vi "ERR Error Dialog.vi"(0 "Error Item":string, 9 "Description":string, 11 "Error In (no error)":errorcluster) -> ()   [LabVIEW 2011]
doc: "This is a 3-button dialog for the use of error handling such that a choice can be made by the user to either Recover from an error, pass the error through, or stop LabVIEW.\n\nThis vi was created by David Gianetto, contact me with any problems, questions, etc."
panel:
  out "Description Display":string
  in  "OK":bool
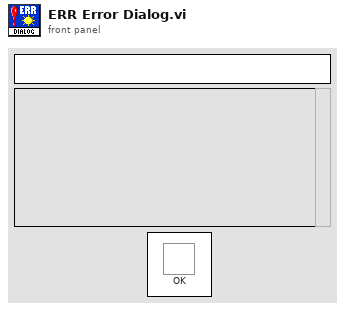
[diagram p1: front panel]
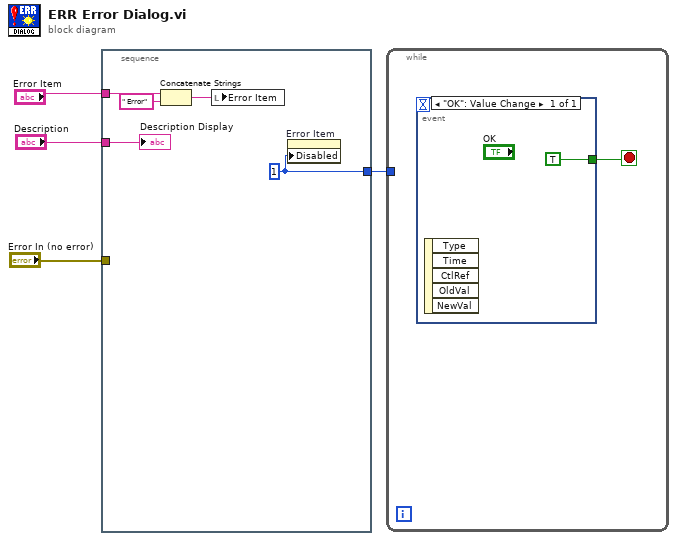
[diagram p0: block diagram]
diagram:
  n1 = stacked-sequence {
    tunnel: [w9] -> w4
    tunnel: "Error In (no error)" -> [_]
    tunnel: "Error Item" -> [w8]
    tunnel: "Description" -> [w5]
    frame #0 {
      w9 = u8 1 ("Disabled")
      n2 = Concatenate Strings(w8, " Error" ("Substring")) -> (w6:string)
      n3 = local write "Error Item"(w6) -> ()
      n4 = property on="Error Item" class="Str"("Disabled"=w9) -> ()  [unwired: 2 in, 2 out]
      "Description Display" <- w5
    }
  }
  n5 = while {
    tunnel: w4 -> [_]
    stop <- w10 stop-if-true
    n6 = event shown="[0] \"OK\": Value Change" {
      selector: _ -> [_]
      dyn-events: _ -> [_]
      timeout: _ -> [_]
      tunnel: [TRUE] -> w10
      event "OK": Value Change {
        n7 = event-data() -> ()  [unwired: 6 out]
      }
    }
  }
